vi "Get Subpanel Status.vi"(0 "GUI Container in":refnum<class "GUI Container.lvclass">, 7 "Subpanel":string, 11 "error in (no error)":errorcluster) -> (4 "GUI Container out":refnum<class "GUI Container.lvclass">, 6 "Subpanel Status":T1, 8 "Subpanel Found":bool, 15 "error out":errorcluster)   [LabVIEW 2023, in "GUI Views.lvlib" / "GUI Container.lvclass"]
uses:
  GUI Container.lvclass
  typedefs/Subpanel Status.ctl
  GUI Container.lvclass/GUI Container.ctl
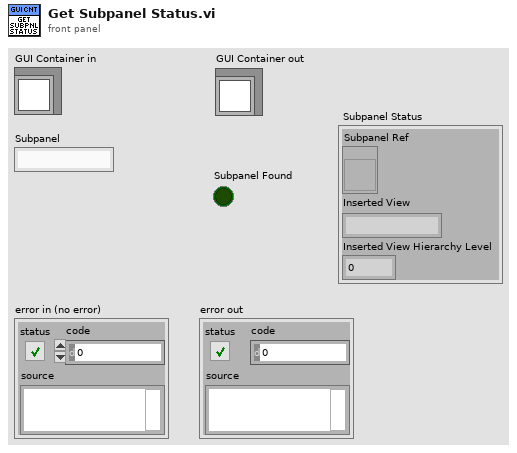
[diagram p1: front panel]
types:
  T1 = typedef "GUI Views.lvlib/GUI Container.lvclass/Subpanel Status.ctl" = cluster{"Subpanel Ref":refnum<vi>, "Inserted View":string, "Inserted View Hierarchy Level":i32}
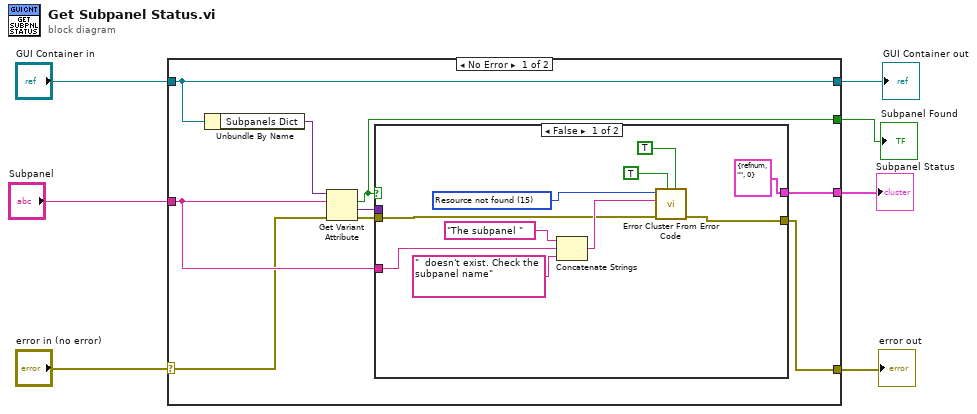
[diagram p0: block diagram]
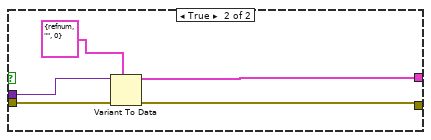
[diagram p2: hidden frame]
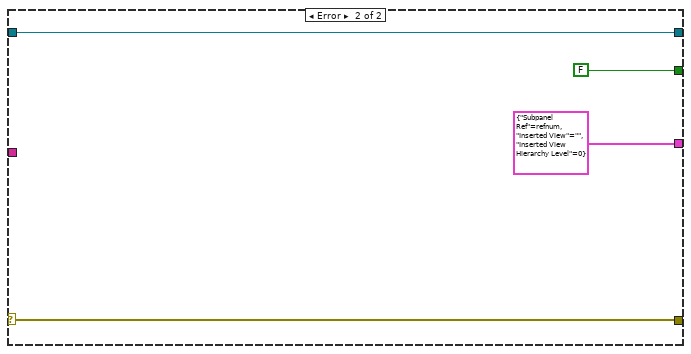
[diagram p3: hidden frame]
diagram:
  n1 = case shown="No Error" "error in (no error)" {
    selector: "error in (no error)" -> [w13 w34]
    tunnel: [w16 w34] -> w7
    tunnel: "GUI Container in" -> [w14 w35]
    tunnel: "Subpanel" -> [w15 _]
    tunnel: [w14 w35] -> w3
    tunnel: [w9 T1 {"Subpanel Ref"=refnum, "Inserted View"="", "Inserted View Hierarchy Level"=0} ("Subpanel Status")] -> w2
    tunnel: [w8 FALSE] -> w1
    frame No Error {
      n2 = Unbundle By Name(w14) -> ("Subpanels Dict"=w12:variant)
      n3 = Get Variant Attribute(Variant=w12, name=w15, error in=w13) -> (found=w8:bool, value=w10:variant, error out=w11:errorcluster)  [unwired: 1 in, 1 out]
      n4 = case shown="False" w8 {
        tunnel: w11 -> [w18 w31]
        tunnel: w10 -> [_ w30]
        tunnel: [w17 w29] -> w16
        tunnel: w15 -> [w24 _]
        tunnel: [T1 {"Subpanel Ref"=refnum, "Inserted View"="", "Inserted View Hierarchy Level"=0} ("Subpanel Status") w28] -> w9
        frame False {
          w19 = 15 items=["No error", "Argument error", "Memory is full", "Out of zone", "End of file", "File already open", "Generic file I/O error", "File not found", "File permission error", "Disk is full", "Duplicate path", "Too many files open", "System feature not enabled", "Resource file not found", "Cannot add resource", "Resource not found", "Image not found", "Image memory error", "Pen does not exist", "Config type invalid", "Config token not found", "Config parse error", "Config memory error", "Bad external code format", "Bad external code offset", "External code not present", "Null window", "Destroy window error", "Null menu", "Print aborted", "Bad print record", "Print driver error", "Windows error during printing", "Memory error during printing", "Print dialog error", "Generic print error", "Invalid device refnum", "Device not found", "Device parameter error", "Device unit error", "Cannot open device", "Device call aborted", "Generic error", "Cancelled by user", "Object ID too low", "Object ID too high", "Object not in heap", "Unknown heap", "Unknown object (invalid DefProc)", "Unknown object (DefProc not in table)", "Message out of range", "Invalid (null) method", "Unknown message", "Manager call not supported", "Bad address", "Network operation in progress", "Network operation timed out", "Connection is busy", "Network attribute not supported", "Network error", "Address in use", "System out of memory", "Connection aborted", "Connection refused", "Not connected", "Already connected", "Connection closed", "Initialization error (interapplication manager)", "Bad occurrence", "Wait on unbound occurrence handler", "Occurrence queue overflow", "Datalog type conflict", "Unused", "Unrecognized type (interapplication manager)", "Memory corrupt", "Failed to make temporary DLL", "Old CIN version", "Drag socket not found", "Failed to load drop-object", "Failed to register OLE object", "Failed to release OLE object", "Format specifier type mismatch", "Unknown format specifier", "Too few format specifiers", "Too many format specifiers", "Scan failed", "Newer CIN version", "Error converting to variant", "Runtime menu error", "Password tampered", "Variant attribute not found", "Incompatible variant data type", "Event data is not available", "Event Store is not present", "Occurrence is not found", "Event Queue is not created", "Event info is not available", "Refnum passed is NULL", "Error retrieving Class GUID", "Error retrieving CoClass GUID", "Error retrieving TypeLib GUID.", "Bad built application magic bytes.", "Specific driver is different from the specific driver associated with the Logical Name.", "There is no session opened to the class driver.", "Max Error", "MAX - Error with config objects", "MAX - Error loading configuration", "MAX - Group not supported"]
          n5 = Concatenate Strings("The subpanel " ("String to Prepend to source (\"\")"), w24, "  doesn't exist. Check the subpanel name" ("string")) -> (w20:string)
          n6 = call <vilib>:"Error Cluster From Error Code.vi"("is warning? (False)"=TRUE, "show call chain? (False)"=TRUE, "error in (no error)"=w18, "error message (\"\")"=w20, "error code (0)"=w19) -> ("error out"=w17:errorcluster)  [unwired: 4 in]
        }
        frame True {
          n7 = Variant To Data(error in=w31, type=T1 {"Subpanel Ref"=refnum, "Inserted View"="", "Inserted View Hierarchy Level"=0} ("Subpanel Status"), Variant=w30) -> (data=w28:T1, error out=w29:errorcluster)
        }
      }
    }
    frame Error {
    }
  }
  "error out" <- w7
  "GUI Container out" <- w3
  "Subpanel Found" <- w1
  "Subpanel Status" <- w2
